vi "CreateCameraGrabQueues.vi"(11 "Framerate (Hz)":i32) -> (0 "Camera state (out)":variant, 1 "VI refs.Grab":T1, 2 "GrabControlQueue":refnum<queue>, 3 "CameraOutQueue":refnum<queue>)   [LabVIEW 2011]
uses:
  CIGrabControlMsg.ctl
  CIGrabControlMsgEnum.ctl
  Typedefs/CmdData_NewFrame.ctl
  <vilib>/vision/Image Controls.llb/IMAQ Image.ctl
  Typedefs/CmdEnum_CameraFrameType.ctl
  Modules/CameraInterface/CIGrabType.ctl
  GlobalVariables.vi
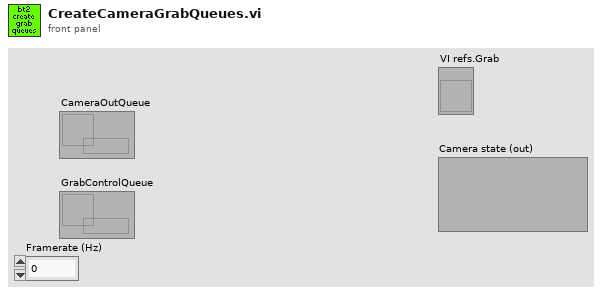
[diagram p1: front panel]
types:
  T1 = typedef "CIGrabType.ctl" = refnum<vi>
  T2 = typedef "CIGrabControlMsg.ctl" = cluster{"Msg":T3}
  T3 = typedef "CIGrabControlMsgEnum.ctl" = enum16{"Stop", "EnableTracking", "DisableTracking"}
  T4 = typedef "CmdData_NewFrame.ctl" = cluster{"Buffer Image":T5, "Frame #":i32, "Hardware ROI Index":i32, "Timestamp":dbl, "Type":T6}
  T5 = typedef "IMAQ Image.ctl" = refnum<image>
  T6 = typedef "CmdEnum_CameraFrameType.ctl" = enum16{"Full", "HardwareROI", "EndGrabMarker"}
  T7 = typedef "CameraInstance.ctl" = cluster{"VI refs":T8, "Camera state":variant}
  T8 = typedef "CameraInterface.ctl" = cluster{"Close":T9, "Get/Set generic config":T10, "Grab":T1, "Show Settings Dialog":T11, "AdjustBeadPos":T12, "Save/load camera settings":T13}
  T9 = typedef "CICloseType.ctl" = refnum<vi>
  T10 = typedef "CIGetSetGenericConfig.ctl" = refnum<vi>
  T11 = typedef "CISettingsDlg.ctl" = refnum<vi>
  T12 = typedef "CIAdjustBeadPos.ctl" = refnum<vi>
  T13 = typedef "CISaveLoadSettings.ctl" = refnum<vi>
  T14 = typedef "GenericCameraConfigType.ctl" = cluster{"Framerate (Hz)":i32, "Exposure time (us)":i32, "Image size":cluster{"Width":i32, "Height":i32}, "Number of buffers":i32}
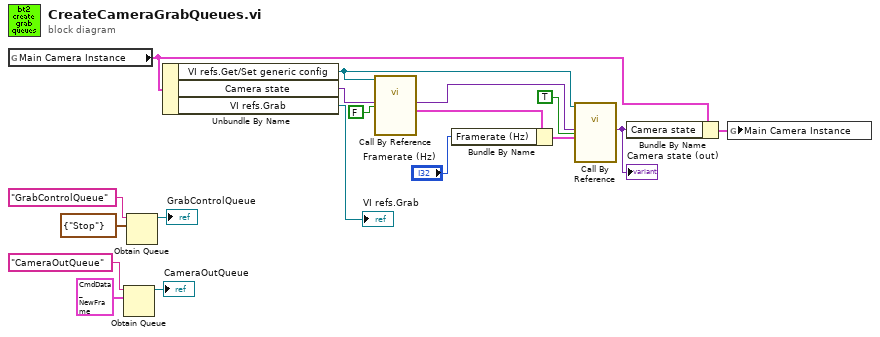
[diagram p0: block diagram]
diagram:
  n1 = global read "GlobalVariables.vi" "Main Camera Instance"() -> (w12:T7)
  n2 = Obtain Queue(name (unnamed)="CameraOutQueue", element data type=T4 {"Buffer Image"=refnum, "Frame #"=0, "Hardware ROI Index"=0, "Timestamp"=0.0, "Type"=enum."Full"} ("Cluster")) -> (queue out=→"CameraOutQueue":refnum<queue>)  [unwired: 3 in, 2 out]
  n3 = Obtain Queue(name (unnamed)="GrabControlQueue", element data type=T2 {"Msg"=enum."Stop"} ("GrabControlMsg")) -> (queue out=→"GrabControlQueue":refnum<queue>)  [unwired: 3 in, 2 out]
  n4 = Unbundle By Name(w12) -> ("VI refs.Get/Set generic config"=w8:T10, "Camera state"=w6:variant, "VI refs.Grab"=→"VI refs.Grab":T1)
  n5 = call-by-ref "?"(reference=w8, "Set? (F)"=FALSE, "Camera state"=w6) -> ("GenericCameraConfig (out)"=w4:T14, "Camera state (out)"=w5:variant)  [unwired: 9 in, 2 out]
  n6 = Bundle By Name(cluster=w4, "Framerate (Hz)"="Framerate (Hz)") -> (w2:T14)
  n7 = call-by-ref "?"(reference=w8, "Set? (F)"=TRUE, "GenericCameraConfig"=w2, "Camera state"=w5) -> ("Camera state (out)"=w11:variant)  [unwired: 8 in, 3 out]
  "Camera state (out)" <- w11
  n8 = Bundle By Name(cluster=w12, "Camera state"=w11) -> (w9:T7)
  n9 = global write "GlobalVariables.vi" "Main Camera Instance"(w9) -> ()
